vi "Destroy.vi"(8 "error in (no error)":errorcluster) -> (0 "error out":errorcluster)   [LabVIEW 2020, in "Global_logger.lvlib"]
uses:
  Global_logger.lvlib
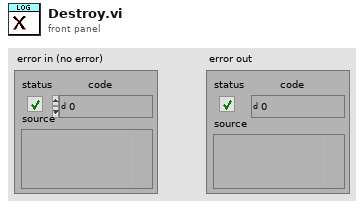
[diagram p1: front panel]
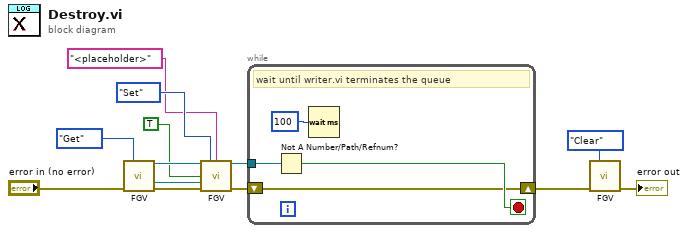
[diagram p0: block diagram]
diagram:
  n1 = call "FGV.vi"("Action"=enum16{"Get", "Set"}."Get", "error in (no error)"="error in (no error)") -> ("queue out"=w12:refnum<queue>, "Writer ref out"=w10:refnum<vi>, "error out"=w9:errorcluster)  [unwired: 8 in, 3 out]
  n2 = call "FGV.vi"("queue in"=w12, "Action"=enum16{"Get", "Set"}."Set", "Logger Name"="<placeholder>", "Destroy Logger in"=TRUE, "Writer ref in"=w10, "error in (no error)"=w9) -> ("queue out"=w7:refnum<queue>, "error out"=w4:errorcluster)  [unwired: 4 in, 4 out]
  n3 = while {
    tunnel: w7 -> [w16]
    shift-right: [w14] -> w3
    shift-left: w4 -> [w14]
    stop <- w15 stop-if-true
    # "wait until writer.vi terminates the queue"
    n4 = Not A Number/Path/Refnum?(number/path/refnum=w16) -> (NaN/Path/Refnum?=w15:bool)
    n5 = Wait (ms)(milliseconds to wait=u32 100) -> ()  [unwired: 1 out]
  }
  n6 = call "FGV.vi"("Action"=enum16{"Get", "Set", "Clear"}."Clear", "error in (no error)"=w3) -> ("error out"=→"error out":errorcluster)  [unwired: 8 in, 5 out]
